vi "Find Size.vi"(8 "error in (no error)":errorcluster, 10 "p":i32, 11 "TeamEffort in":refnum<class "TeamEffort.lvclass">=refnum) -> (0 "error out":errorcluster, 1 "Direction":T1, 2 "Action":T2, 3 "TeamEffort out":refnum<class "TeamEffort.lvclass">)   [LabVIEW 2014, in "TeamEffort.lvclass"]
uses:
  Square/Shawn/TeamEffort/TeamEffort.lvclass
  SquareBattle Arena/Direction Enum.ctl
  SquareBattle Arena/SquareBattle Arena.lvclass
  SquareBattle Arena/Action Enum.ctl
panel:
  in  "Maze (0: Empty, -1: Enemy. >0: Teammate":i32[][](array[numeric])
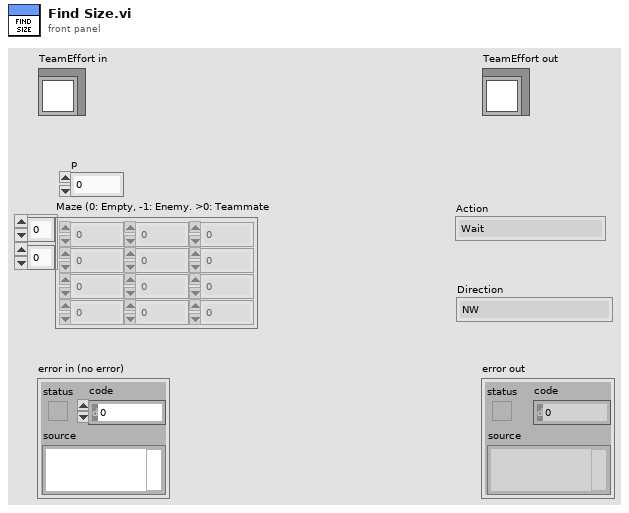
[diagram p1: front panel]
types:
  T1 = typedef "SquareBattle Arena.lvlib/SquareBattle Arena.lvclass/Direction Enum.ctl" = enum16{"NW", "N", "NE", "E", "SE", "S", "SW", "W"}
  T2 = typedef "SquareBattle Arena.lvlib/SquareBattle Arena.lvclass/Action Enum.ctl" = enum16{"Wait", "Move", "Attack", "Replicate"}
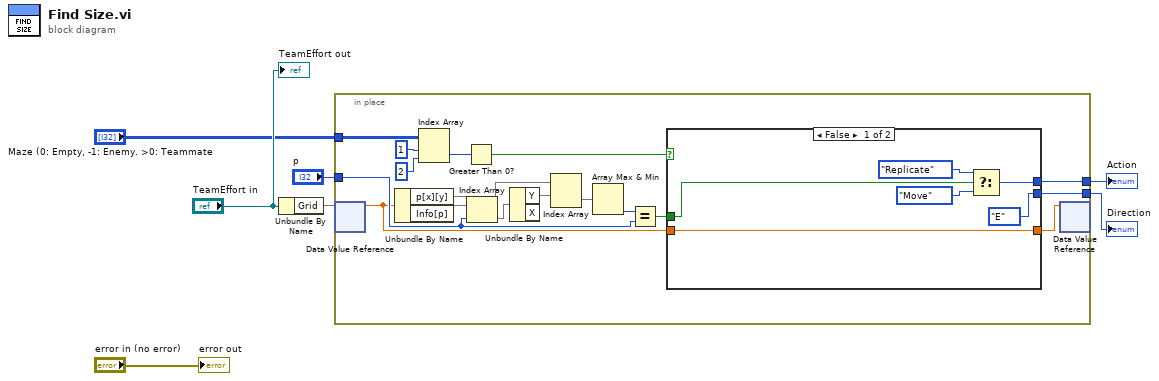
[diagram p0: block diagram]
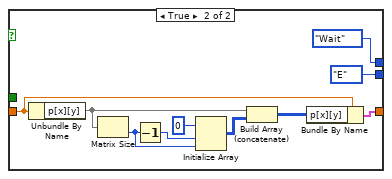
[diagram p2: hidden frame]
diagram:
  n1 = Unbundle By Name("TeamEffort in") -> ("Grid"=w7)
  n2 = in-place {
    in-place-border: "p" -> [w18]
    in-place-border: "Maze (0: Empty, -1: Enemy. >0: Teammate" -> [w17]
    in-place-border: [w11] -> w2
    in-place-border: [w10] -> w1
    n3 = in-place-dvr #1(w7) -> (w9:dbl)  [unwired: 1 out]
    n4 = Unbundle By Name(w9) -> ("p[x][y]"=w22, "Info[p]"=w24)
    n5 = Index Array(array=w17, index (row)=1, index (col)=2 ("index (row)")) -> (element=w14:i32)
    n6 = Greater Than 0?(x=w14) -> (x > 0?=w13:bool)
    n7 = Index Array(array=w24, index=w18) -> (element=w23)
    n8 = Unbundle By Name(w23) -> ("Y"=w21)  [unwired: 1 out]
    n9 = Index Array(array=w22, index (row)=w21) -> (element=w20)  [unwired: 1 in]
    n10 = Array Max & Min(array=w20) -> (min index (indices)=w19:i32)  [unwired: 3 out]
    n11 = Equal?(x=w19, y=w18) -> (x = y?=w12:bool)
    n12 = case shown="False" w13 {
      tunnel: w12 -> [w30 _]
      tunnel: [Direction_Enum."E" ("Direction") Direction_Enum."E" ("Direction")] -> w11
      tunnel: [w26 Action_Enum."Wait" ("Action")] -> w10
      tunnel: w9 -> [w25 w35]
      tunnel: [w25 w33] -> w8
      frame False {
        n13 = Select(t=Action_Enum."Replicate" ("Action"), s=w30, f=Action_Enum."Move" ("Action")) -> (s? t:f=w26:T2)
      }
      frame True {
        n14 = Unbundle By Name(w35) -> ("p[x][y]"=w39)
        n15 = Matrix Size(0:w39) -> (2:w38:i32)  [unwired: 1 out]
        n16 = Decrement(x=w38) -> (x-1=w37:i32)
        n17 = Initialize Array(0, w37, w38) -> (w36:i32[][])
        n18 = Build Array (concatenate)(w39, w36) -> (w34:i32[][])
        n19 = Bundle By Name(cluster=w35, "p[x][y]"=w34) -> (w33:cluster{})
      }
    }
    n20 = in-place-dvr #1(w8) -> ()  [unwired: 2 out]
  }
  "Action" <- w1
  "Direction" <- w2
  "error out" <- "error in (no error)"
  "TeamEffort out" <- "TeamEffort in"
